vi "Write Timeout.vi"(8 "error in (no error)":errorcluster, 10 "Timeout":i32=-1, 11 "bt_Synch in":refnum<class "bt_WaitOn_Synch.lvclass">) -> (0 "error out":errorcluster, 3 "bt_Synch out":refnum<class "bt_WaitOn_Synch.lvclass">)   [LabVIEW 2021, in "BT.lvlib" / "bt_WaitOn_Synch.lvclass"]
uses:
  bt_WaitOn_Synch.lvclass
  bt_WaitOn_Synch.lvclass/bt_WaitOn_Synch.ctl
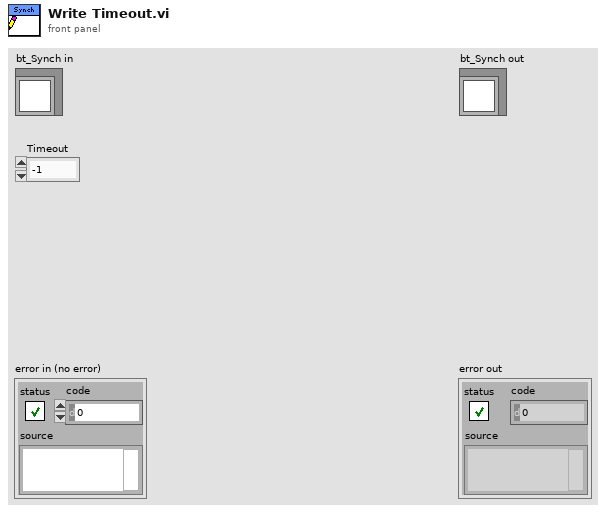
[diagram p1: front panel]
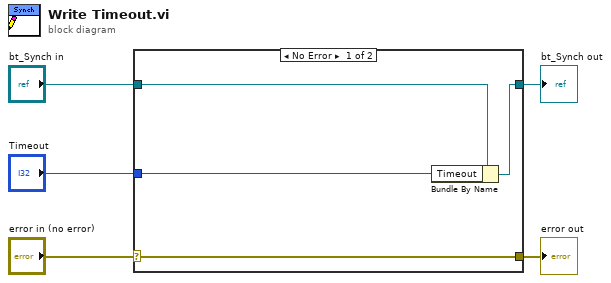
[diagram p0: block diagram]
diagram:
  n1 = case shown="No Error" "error in (no error)" {
    selector: "error in (no error)" -> [w9 w10]
    tunnel: [w9 w10] -> w4
    tunnel: [w7 w11] -> w2
    tunnel: "bt_Synch in" -> [w8 w11]
    tunnel: "Timeout" -> [w6 _]
    frame No Error {
      n2 = Bundle By Name(cluster=w8, "Timeout"=w6) -> (w7:refnum<class "bt_WaitOn_Synch.lvclass">)
    }
    frame Error {
    }
  }
  "error out" <- w4
  "bt_Synch out" <- w2
